vi "editGoalAmount.vi"(8 "error in (no error)":errorcluster, 11 "Goal in":refnum<class "Goal.lvclass">) -> (0 "error out":errorcluster, 2 "UserConfirm?":bool, 3 "Goal out":refnum<class "Goal.lvclass">)   [LabVIEW 2020, in "Goal.lvclass"]
uses:
  Goal.lvclass
  UserEditableAmount/UserEditableAmount.lvclass
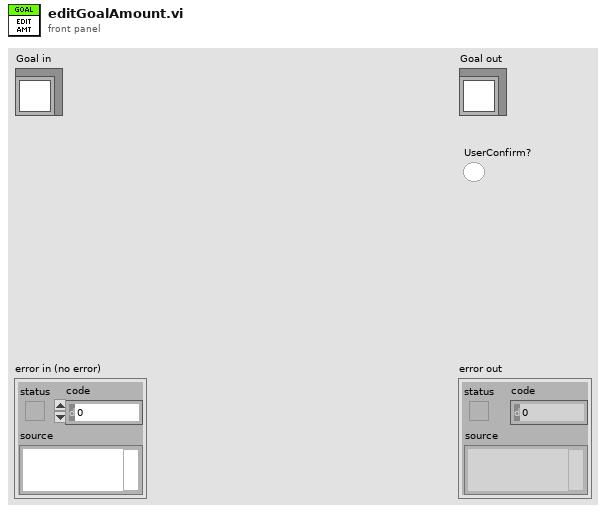
[diagram p1: front panel]
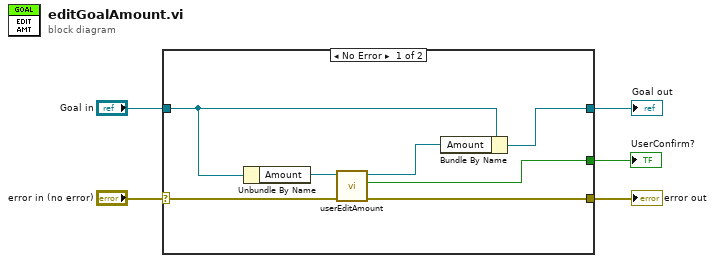
[diagram p0: block diagram]
diagram:
  n1 = case shown="No Error" "error in (no error)" {
    selector: "error in (no error)" -> [w7 w14]
    tunnel: [w6 w14] -> w4
    tunnel: [w9 w13] -> w2
    tunnel: "Goal in" -> [w11 w13]
    tunnel: [w8 _] -> w1
    frame No Error {
      n2 = Unbundle By Name(w11) -> ("Amount"=w12:refnum<class "UserEditableAmount.lvclass">)
      n3 = call "userEditAmount.vi"("error in (no error)"=w7, "UserEditableAmount.lvclass"=w12) -> ("error out"=w6:errorcluster, "UserConfirm?"=w8:bool, "UserEditableAmount.lvclass"=w10:refnum<class "UserEditableAmount.lvclass">)  [unwired: 7 in]
      n4 = Bundle By Name(cluster=w11, "Amount"=w10) -> (w9:refnum<class "Goal.lvclass">)
    }
    frame Error {
    }
  }
  "error out" <- w4
  "Goal out" <- w2
  "UserConfirm?" <- w1
